vi "RSZVB Setup Recall.vi"(8 "error in (no error)":errorcluster {"code" format="%.0x"}, 10 "File Name (setup.zvx)":string="setup.zvx", 11 "VISA session":refnum<visa-resource-name>) -> (0 "error out":errorcluster {"code" format="%.0x"}, 3 "dup VISA session":refnum<visa-resource-name>)   [LabVIEW 2011]
doc: "This VI loads configuration data from a specified setup file and sets the analyzer to the corresponding instrument state.\n\nRemote-control command(s):\nMMEMory:LOAD:STATe <numeric_value>,'<file_name>'"
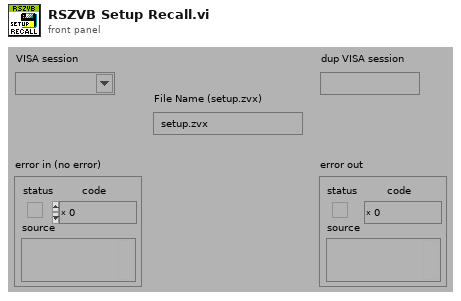
[diagram p1: front panel]
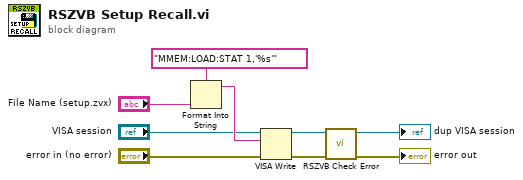
[diagram p0: block diagram]
diagram:
  n1 = Format Into String(format string="MMEM:LOAD:STAT 1,'%s'", "File Name (setup.zvx)") -> (resulting string=w6:string)  [unwired: 2 in, 1 out]
  n2 = VISA Write(VISA resource name="VISA session", write buffer=w6, error in (no error)="error in (no error)") -> (VISA resource name out=w9:refnum<visa-resource-name>, error out=w8:errorcluster)  [unwired: 1 out]
  n3 = call "RSZVB Check Error.vi"("error in (no error)"=w8, "VISA session"=w9) -> ("error out"=→"error out":errorcluster, "dup VISA session"=→"dup VISA session":refnum<visa-resource-name>)  [unwired: 8 in]
